vi "Inject.vi"(8 "error in (no error)":errorcluster, 9 "Injection Data":variant, 10 "Internal Message Queue":refnum<queue>, 11 "TestProcessor in":refnum<class "TestProcessor.lvclass">) -> (0 "error out":errorcluster, 3 "TestProcessor out":refnum<class "TestProcessor.lvclass">)   [LabVIEW 2023, in "HAF.lvlib" / "TestProcessor.lvclass"]
doc: "Add the Command Directors passed in the Message Data to the current set of Command Directors for processing."
uses:
  TestProcessor.lvclass
  TestProcessor.lvclass/TestProcessor.ctl
  CommandDirector/CommandDirector.lvclass
  Injection Data.ctl
  All Internal Message Ids.ctl
  HAF.lvlib
  Message.ctl
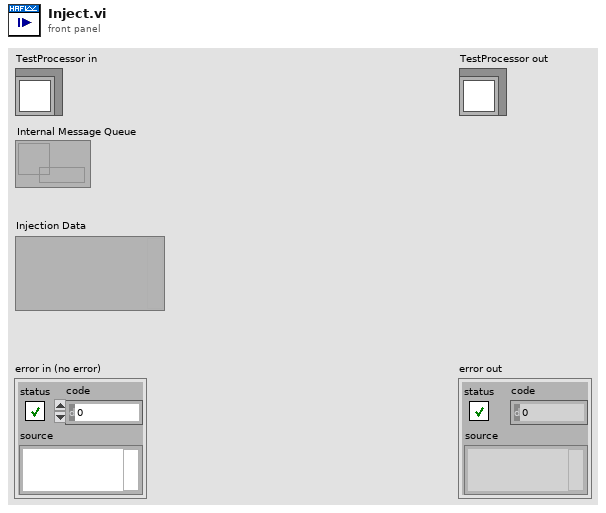
[diagram p1: front panel]
types:
  T1 = typedef "HAF.lvlib/All Internal Message Ids.ctl" = cluster{"Initialise":string, "Process":string, "Continue":string, "Done":string, "Pause":string, "Resume":string, "Stop":string, "Exit":string, "Inject":string}
  T2 = typedef "Injection Data.ctl" = cluster{"Command Directors":refnum<class "CommandDirector.lvclass">[], "Wait Time":u32}
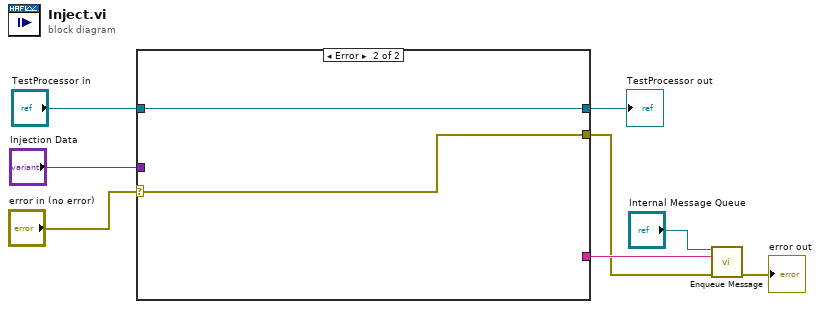
[diagram p0: block diagram]
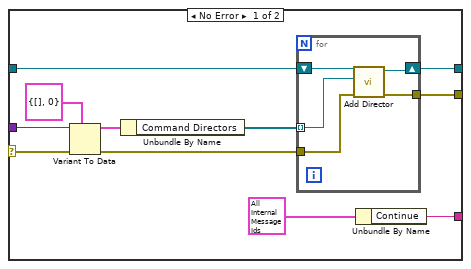
[diagram p2: hidden frame]
diagram:
  n1 = case shown="Error" "error in (no error)" {
    selector: "error in (no error)" -> [w18 w26]
    tunnel: [w9 w26] -> w2
    tunnel: [w12 w25] -> w6
    tunnel: "TestProcessor in" -> [w14 w25]
    tunnel: "Injection Data" -> [w19 _]
    tunnel: [w10 _] -> w3
    frame No Error {
      n2 = Variant To Data(error in=w18, type=T2 {"Command Directors"=[], "Wait Time"=0} ("Injection Data"), Variant=w19) -> (data=w16:T2, error out=w13:errorcluster)
      n3 = Unbundle By Name(w16) -> ("Command Directors"=w15:refnum<class "CommandDirector.lvclass">[])
      n4 = for {
        tunnel: w15 -> [w23] mode=indexing
        tunnel: w13 -> [w22]
        shift-right: [w21] -> w12
        shift-left: w14 -> [w24]
        tunnel: [w20] -> w9
        n5 = call-dynamic "Add Director.vi"("error in (no error)"=w22, "Command Director"=w23, "TestProcessor in"=w24) -> ("error out"=w20:errorcluster, "TestProcessor out"=w21:refnum<class "TestProcessor.lvclass">)  [unwired: 7 in]
      }
      n6 = Unbundle By Name(T1 {"Initialise"="Initialise", "Process"="Process", "Continue"="Continue", "Done"="Done", "Pause"="Pause", "Resume"="Resume", "Stop"="Stop", "Exit"="Exit", "Inject"=""} ("Message Ids")) -> ("Continue"=w10:string)
    }
    frame Error {
    }
  }
  "TestProcessor out" <- w6
  n7 = call "Enqueue Message.vi"("Message Queue In"="Internal Message Queue", "Message Id"=w3, "error in (no error)"=w2) -> ("error out"=→"error out":errorcluster)  [unwired: 11 in, 1 out]
